vi "Jet_GUI.vi"() -> ()   [LabVIEW 2020]
uses:
  Shared/GUI_Template/GUI_master/tcp new data cluster.ctl
  Shared/GUI_Template/GUI_master/tcp_new_data_event.ctl
panel:
  in  "stop":bool
  in  "Tab Control":enum32{"Hi P Cntlr", "Med P Cntlr"}(tab)
  in  "set pressure::3":dbl caption="Hi Press. Set [PSIG]" min=0.0 max=600.0 format="%.1f"
  in  "read pressure::3":dbl caption="Hi Press. Read [PSIG]" min=0.0 max=0.0 format="%.1f"
  in  "set pressure::9":dbl caption="Med. Press. Set [PSIG]" min=0.0 max=150.0 format="%.1f"
  in  "read pressure::9":dbl caption="Med. Press. Read [PSIG]" min=0.0 max=0.0 format="%.1f"
  out "GUIdevice 9":string="StagingMedPController"
  in  "Save::2":bool caption="Save"
  in  "trigger::2":bool caption="Trig"
  out "AI_array.Channel 0::2":waveform(dbl)[](graph) caption="Jet Voltage trace"
  out "GUIdevice 8":string="StagingLowPressure2"
  out "GUIdevice 7":string="StagingDischargeHV"
  out "GUIdevice 6":string="StagingLowPressure1"
  in  "reading.var 28::4":dbl caption="SAC3 Convec" min=-100000.0 max=100000.0 format="%#_6e"
  in  "Delay.Ch C::5":dbl=0.042 caption="Jet Delay [s]" min=-0.1 max=0.1 format="%.5f"
  out "GUIdevice 5":string="StagingDG645_2"
  in  "reading.var 4::4":dbl caption="SAC3 Ion" min=-100000.0 max=100000.0 format="%_4e"
  out "GUIdevice 4":string="DS-A-Cave_VacSys_Feedback_Double"
  in  "DigitalOutput.Channel 2::2":bool caption="Exhaust Valve"
  in  "Link.com2::1":string caption="Jet Trigger status"
  in  "Jet Trigger":bool caption="Jet Trig"
  out "GUIdevice 3":string="StagingHighPressureController"
  out "GUIdevice 2":string="Staging_USB6210_1"
  out "GUIdevice 1":string="StagingNISwitch"
  out "tcp data event":T1
  out "error IO 2":errorcluster
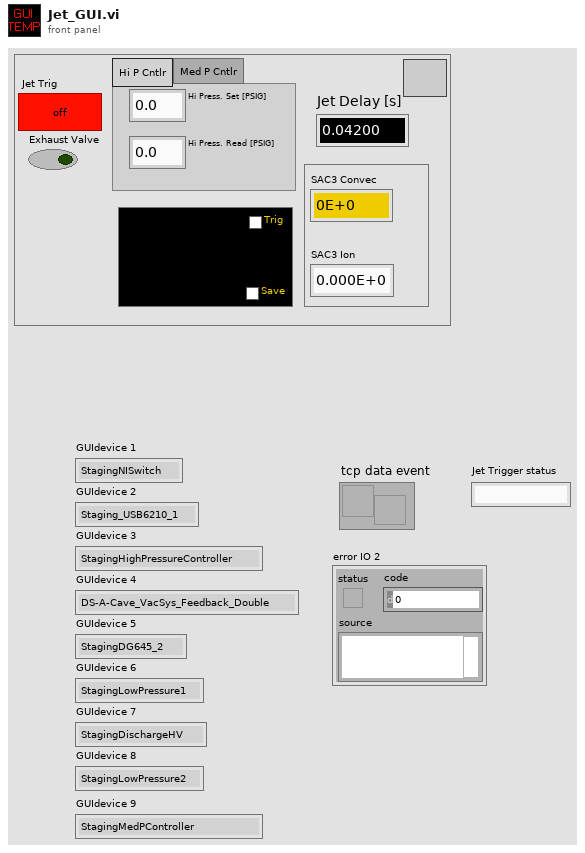
[diagram p1: front panel]
types:
  T1 = typedef "tcp_new_data_event.ctl" = refnum<user-event>
  T2 = typedef "tcp new data cluster.ctl" = cluster{"EventEnum":enum16{"new data", "connection status update"}, "Device name":string}
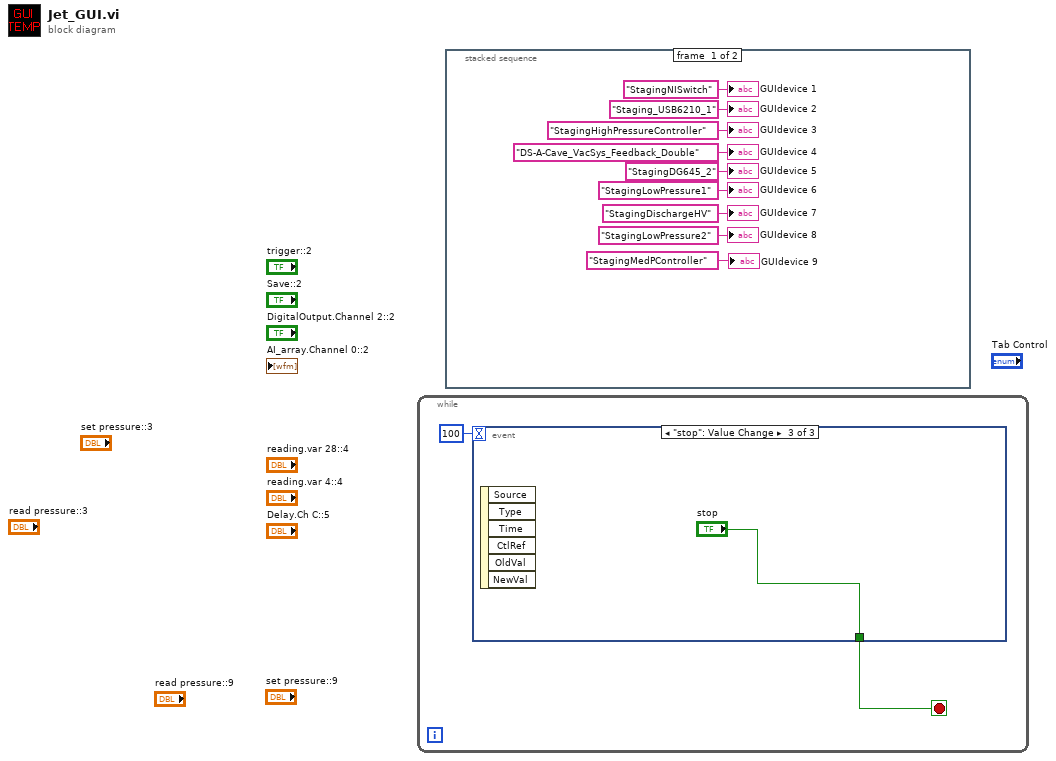
[diagram p0: block diagram]
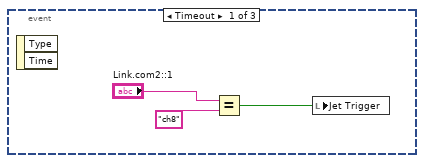
[diagram p2: hidden frame]
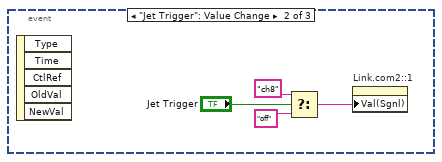
[diagram p3: hidden frame]
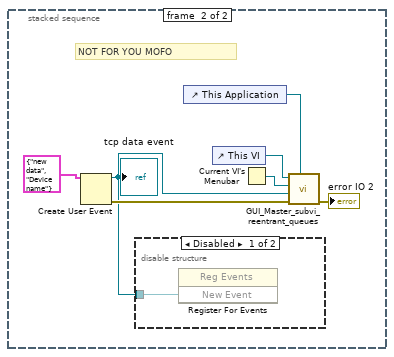
[diagram p4: hidden frame]
diagram:
  n1 = while {
    stop <- w2 stop-if-true
    n2 = event shown="[2] \"stop\": Value Change" {
      selector: _ -> [_ _ _]
      dyn-events: _ -> [_ _ _]
      timeout: 100 -> [_ _ _]
      tunnel: [_ _ "stop"] -> w2
      event Timeout {
        n3 = event-data() -> ()  [unwired: 1 in, 2 out]
        n4 = Equal?(x="Link.com2::1", y="ch8") -> (x = y?=w4:bool)
        n5 = local write "Jet Trigger"(w4) -> ()
      }
      event "Jet Trigger": Value Change {
        n6 = event-data() -> ()  [unwired: 1 in, 5 out]
        n7 = Select(t="ch8", s="Jet Trigger", f="off") -> (s? t:f=w6:string)
        n8 = property on="Link.com2::1" class="Str"("Val(Sgnl)"=w6) -> ()  [unwired: 2 in, 2 out]
      }
      event "stop": Value Change {
        n9 = event-data() -> ()  [unwired: 1 in, 6 out]
      }
    }
  }
  n10 = stacked-sequence {
    frame #0 {
      "GUIdevice 1" <- "StagingNISwitch" ("GUIdevice 1")
      "GUIdevice 2" <- "Staging_USB6210_1" ("GUIdevice 2")
      "GUIdevice 3" <- "StagingHighPressureController" ("GUIdevice 3")
      "GUIdevice 4" <- "DS-A-Cave_VacSys_Feedback_Double" ("GUIdevice 4")
      "GUIdevice 5" <- "StagingDG645_2" ("GUIdevice 5")
      "GUIdevice 6" <- "StagingLowPressure1" ("GUIdevice 6")
      "GUIdevice 7" <- "StagingDischargeHV" ("GUIdevice 23")
      "GUIdevice 8" <- "StagingLowPressure2" ("GUIdevice 6")
      "GUIdevice 9" <- "StagingMedPController" ("GUIdevice 6")
    }
    frame #1 {
      # "NOT FOR YOU MOFO"
      n11 = Create User Event(user event datatype=T2 {"EventEnum"=enum."new data", "Device name"="Device name"} ("New Event")) -> (user event=w21:refnum<user-event>, error out=w22:errorcluster)  [unwired: 1 in]
      "tcp data event" <- w21
      n12 = disable-structure shown="Disabled" {
        disable-tunnel: w21 -> [w27 _]
        frame Disabled {
          n13 = register-events(w27) -> ()  [unwired: 2 in, 2 out]
        }
        frame Enabled {
        }
      }
      n14 = control-ref of="This Application"() -> (w20:refnum<vi>)
      n15 = control-ref of="This VI"() -> (w25:refnum<vi>)
      n16 = Current VI's Menubar() -> (w24:refnum<k9>)
      n17 = call "GUI_Master_subvi_reentrant_queues.vi"("This Application"=w20, "error in (no error)"=w22, "tcp data event"=w21, "Caller menu reference"=w24, "Caller VI ref"=w25) -> ("error out"=→"error IO 2":errorcluster)  [unwired: 6 in]
    }
  }
